vi "asset.get[].vi"(8 "error in":errorcluster, 10 "Asset RIDs":string[](array[string]), 11 "Nominal Client in":refnum<class "Nominal Client.lvclass">) -> (0 "error out":errorcluster, 2 "Assets":refnum<class "asset.lvclass">[](array[class]), 3 "Nominal Client out":refnum<class "Nominal Client.lvclass">)   [LabVIEW 2020, in "Nominal Client.lvclass"]
doc: "Triggers an ingest job, allowing either creating a new dataset or uploading to an existing one. This endpoint is meant to supersede all other ingestion endpoints as their functionality gets migrated to this one."
uses:
  Nominal Client.lvclass
  asset/asset.lvclass
  Nominal Client.lvclass/Nominal Client.ctl
  nominal types/workspace/workspace.lvclass/workspace.ctl
  nominal types/workspace/rid.get.vi
  c20a9d0c-990e-4b00-9818-b2ddac785778.vi
  trace.payload_received.vi
  error.vi
  trace.payload_sent.vi
  create.authorization_header.vi
  trace.generate.vi
  trace.calling_method.vi
  error.vi/859f8e04-e495-489b-b5b4-7ac163f56130.vi
  <vilib>/AdvancedString/1D String Array to Delimited String.vi
  <vilib>/JDP Science/JDP Science Common Utilities/Trim Whitespace__JDP.vi
  api_token.get.vi
  <vilib>/JDP Science/JSONtext/Variant to JSON Text.vi
  <vilib>/Utility/libraryn.llb/Get File Extension.vi
  log_file.write.vi
  <vilib>/Utility/error.llb/Error Cluster From Error Code.vi
  <vilib>/JDP Science/JSONtext/JSON text to Variant.vi
  <vilib>/JDP Science/JSONtext/LVClass Serializer/JSONtext LVClass Serializer.lvclass
  <vilib>/addons/_JKI.lib/REST Client/classes/Response Headers/Response Headers.lvclass
  <vilib>/addons/_JKI.lib/REST Client/classes/REST Client/REST Client.lvclass
  <vilib>/JDP Science/JSONtext/JSONtext.lvlib
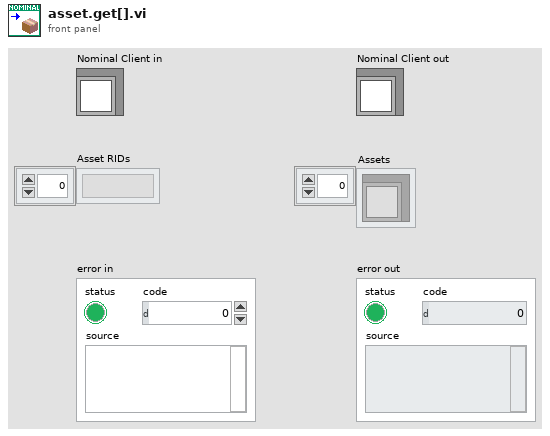
[diagram p1: front panel]
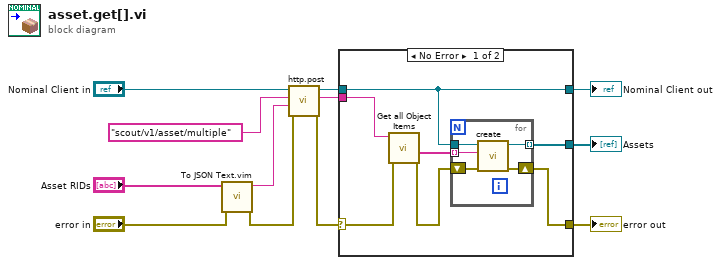
[diagram p0: block diagram]
diagram:
  n1 = call "To JSON Text.vim"("error in (no error)"="error in", "Anything"="Asset RIDs") -> ("error out"=w1:errorcluster, "<JSON>"=w2:string)  [unwired: 8 in]
  n2 = call "http.post.vi"("error in"=w1, "Request body"=w2, "Path"="scout/v1/asset/multiple", "Nominal Client in"="Nominal Client in") -> ("error out"=w6:errorcluster, "Response"=w11:string, "Nominal Client out"=w9:refnum<class "Nominal Client.lvclass">)  [unwired: 4 in, 1 out]
  n3 = case shown="No Error" w6 {
    selector: w6 -> [w13 w26]
    tunnel: w11 -> [w16 _]
    tunnel: w9 -> [w14 w25]
    tunnel: [w14 w25] -> w8
    tunnel: [w19 _] -> w7
    tunnel: [w18 w26] -> w5
    frame No Error {
      n4 = call <vilib>:"Get all Object Items.vi"("error in (no error)"=w13, "JSON"=w16) -> ("error out"=w15:errorcluster, "<JSON>"=w17:string[])  [unwired: 6 in, 2 out]
      n5 = for {
        tunnel: w17 -> [w24] mode=indexing
        tunnel: [w23] -> w19 mode=indexing
        shift-right: [w21] -> w18
        shift-left: w15 -> [w22]
        tunnel: w14 -> [w20]
        n6 = call "create.vi"("error in"=w22, "asset"=w24, "Nominal Client"=w20) -> ("error out"=w21:errorcluster, "asset"=w23:refnum<class "asset.lvclass">)  [unwired: 7 in]
      }
    }
    frame Error {
    }
  }
  "Nominal Client out" <- w8
  "error out" <- w5
  "Assets" <- w7
